vi "Save and Close System Definition.vi"(7 "System Definition Path":path, 8 "error in (no error)":errorcluster, 9 "Target Refnum":refnum<k24>, 10 "Root Refnum":refnum<k24>, 11 "System Definition Refnum":refnum<k24>) -> (0 "error out":errorcluster)   [LabVIEW 2019]
uses:
  NationalInstruments.VeriStand.SystemDefinitionAPI
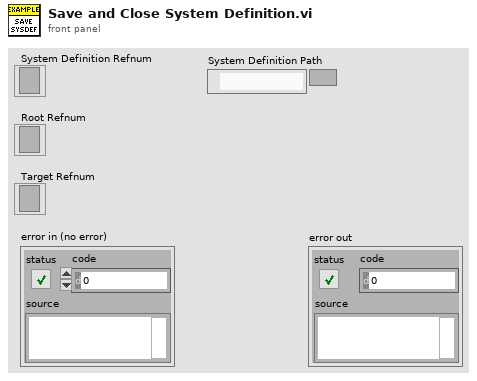
[diagram p1: front panel]
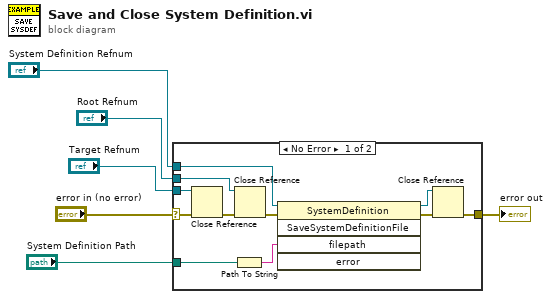
[diagram p0: block diagram]
diagram:
  n1 = case shown="No Error" "error in (no error)" {
    selector: "error in (no error)" -> [w13 w18]
    tunnel: [w7 w18] -> w5
    tunnel: "System Definition Path" -> [w9 _]
    tunnel: "Target Refnum" -> [w12 _]
    tunnel: "Root Refnum" -> [w11 _]
    tunnel: "System Definition Refnum" -> [w10 _]
    frame No Error {
      n2 = Close Reference(reference=w12, error in (no error)=w13) -> (error out=w14:errorcluster)
      n3 = Path To String(path=w9) -> (string=w8:string)
      n4 = Close Reference(reference=w11, error in (no error)=w14) -> (error out=w15:errorcluster)
      n5 = invoke class="SystemDefinition" method="SaveSystemDefinitionFile"(reference=w10, error in=w15, "filepath"=w8) -> (reference out=w17:refnum<k24>, error out=w16:errorcluster)  [unwired: 2 in, 3 out]
      n6 = Close Reference(reference=w17, error in (no error)=w16) -> (error out=w7:errorcluster)
    }
    frame Error {
    }
  }
  "error out" <- w5
